vi "LoopselFF_1_or_2cam_eventdriven_HS.VI"() -> ()   [LabVIEW 2015]
uses:
  board.vis/Globals.vi
  <vilib>/Analysis/NI_AALBase.lvlib
panel:
  in  "ADC mode":enum32{"1", "2", "3"}(radio)=enum."3"
  out "tRMS":dbl=8.272957184592048 format="%0#.1f"
  out "mean":dbl=3064.5285285285286 format="%#_4f"
  in  "rms_pixel":u16=100
  in  "continuous":bool=TRUE
  out "curr.block":u8=1
  out "Measure ON":bool
  in  "Board select\n1: board 1\n2: board 2\n3: both boards":u8=3
  in  "no.of blocks (nob)\npress enter":u32=1
  in  "block":u32(slide)=1 max=10 scale=0.9..1.0
  out "Signalverlaufgraph 2":u16[](graph)=[0, 0, 543, 543, 0, 1, 0, 0, 2, 2, 3, 3, 4, 4, 5, 5, 6, 6, 7, 7, 8, 8, 9, 9, 10, 10, 11, 11, 12, 12, 13, 13, 14, 14, 15, 15, 16, 16, 17, 17, 18, 18, 19, 19, 20, 20, 21, 21, 22, 22, 23, 23, 24, 24, 25, 25, 26, 26, 27, 27, 28, 28, 29, 29, 30, 30, 31, 31, 32, 32, 33, 33, 34, 34, 35, 35, 36, 36, 37, 37, 38, 38, 39, 39, 40, 40, 41, 41, 42, 42, 43, 43, 44, 44, 45, 45, 46, 46, 47, 47, 48, 48, 49, 49, 50, 50, 51, 51, 52, 52, 53, 53, 54, 54, 55, 55, 56, 56, 57, 57, 58, 58, 59, 59, 60, 60, 61, 61, 62, 62, 63, 63, 64, 64, 65, 65, 66, 66, 67, 67, 68, 68, 69, 69, 70, 70, 71, 71, 72, 72, 73, 73, 74, 74, 75, 75, 76, 76, 77, 77, 78, 78, 79, 79, 80, 80, 81, 81, 82, 82, 83, 83, 84, 84, 85, 85, 86, 86, 87, 87, 88, 88, 89, 89, 90, 90, 91, 91, 92, 92, 93, 93, 94, 94, 95, 95, 96, 96, 97, 97, 98, 98, 99, 99, 100, 100, 101, 101, 102, 102, 103, 103, 104, 104, 105, 105, 106, 106, 107, 107, 108, 108, 109, 109, 110, 110, 111, 111, 112, 112, 113, 113, 114, 114, 115, 115, 116, 116, 117, 117, 118, 118, 119, 119, 120, 120, 121, 121, 122, 122, 123, 123, 124, 124, 125, 125, 126, 126, 127, 127, 128, 128, 129, 129, 130, 130, 131, 131, 132, 132, 133, 133, 134, 134, 135, 135, 136, 136, 137, 137, 138, 138, 139, 139, 140, 140, 141, 141, 142, 142, 143, 143, 144, 144, 145, 145, 146, 146, 147, 147, 148, 148, 149, 149, 150, 150, 151, 151, 152, 152, 153, 153, 154, 154, 155, 155, 156, 156, 157, 157, 158, 158, 159, 159, 160, 160, 161, 161, 162, 162, 163, 163, 164, 164, 165, 165, 166, 166, 167, 167, 168, 168, 169, 169, 170, 170, 171, 171, 172, 172, 173, 173, 174, 174, 175, 175, 176, 176, 177, 177, 178, 178, 179, 179, 180, 180, 181, 181, 182, 182, 183, 183, 184, 184, 185, 185, 186, 186, 187, 187, 188, 188, 189, 189, 190, 190, 191, 191, 192, 192, 193, 193, 194, 194, 195, 195, 196, 196, 197, 197, 198, 198, 199, 199, 200, 200, 201, 201, 202, 202, 203, 203, 204, 204, 205, 205, 206, 206, 207, 207, 208, 208, 209, 209, 210, 210, 211, 211, 212, 212, 213, 213, 214, 214, 215, 215, 216, 216, 217, 217, 218, 218, 219, 219, 220, 220, 221, 221, 222, 222, 223, 223, 224, 224, 225, 225, 226, 226, 227, 227, 228, 228, 229, 229, 230, 230, 231, 231, 232, 232, 233, 233, 234, 234, 235, 235, 236, 236, 237, 237, 238, 238, 239, 239, 240, 240, 241, 241, 242, 242, 243, 243, 244, 244, 245, 245, 246, 246, 247, 247, 248, 248, 249, 249, 250, 250, 251, 251, 252, 252, 253, 253, 254, 254, 255, 255, 256, 256, 257, 257, 258, 258, 259, 259, 260, 260, 261, 261, 262, 262, 263, 263, 264, 264, 265, 265, 266, 266, 267, 267, 268, 268, 269, 269, 270, 270, 271, 271, 272, 272, 273, 273, 274, 274, 275, 275, 276, 276, 277, 277, 278, 278, 279, 279, 280, 280, 281, 281, 282, 282, 283, 283, 284, 284, 285, 285, 286, 286, 287, 287, 288, 288, 289, 289, 290, 290, 291, 291, 292, 292, 293, 293, 294, 294, 295, 295, 296, 296, 297, 297, 298, 298, 299, 299, 300, 300, 301, 301, 302, 302, 303, 303, 304, 304, 305, 305, 306, 306, 307, 307, 308, 308, 309, 309, 310, 310, 311, 311, 312, 312, 313, 313, 314, 314, 315, 315, 316, 316, 317, 317, 318, 318, 319, 319, 320, 320, 321, 321, 322, 322, 323, 323, 324, 324, 325, 325, 326, 326, 327, 327, 328, 328, 329, 329, 330, 330, 331, 331, 332, 332, 333, 333, 334, 334, 335, 335, 336, 336, 337, 337, 338, 338, 339, 339, 340, 340, 341, 341, 342, 342, 343, 343, 344, 344, 345, 345, 346, 346, 347, 347, 348, 348, 349, 349, 350, 350, 351, 351, 352, 352, 353, 353, 354, 354, 355, 355, 356, 356, 357, 357, 358, 358, 359, 359, 360, 360, 361, 361, 362, 362, 363, 363, 364, 364, 365, 365, 366, 366, 367, 367, 368, 368, 369, 369, 370, 370, 371, 371, 372, 372, 373, 373, 374, 374, 375, 375, 376, 376, 377, 377, 378, 378, 379, 379, 380, 380, 381, 381, 382, 382, 383, 383, 384, 384, 385, 385, 386, 386, 387, 387, 388, 388, 389, 389, 390, 390, 391, 391, 392, 392, 393, 393, 394, 394, 395, 395, 396, 396, 397, 397, 398, 398, 399, 399, 400, 400, 401, 401, 402, 402, 403, 403, 404, 404, 405, 405, 406, 406, 407, 407, 408, 408, 409, 409, 410, 410, 411, 411, 412, 412, 413, 413, 414, 414, 415, 415, 416, 416, 417, 417, 418, 418, 419, 419, 420, 420, 421, 421, 422, 422, 423, 423, 424, 424, 425, 425, 426, 426, 427, 427, 428, 428, 429, 429, 430, 430, 431, 431, 432, 432, 433, 433, 434, 434, 435, 435, 436, 436, 437, 437, 438, 438, 439, 439, 440, 440, 441, 441, 442, 442, 443, 443, 444, 444, 445, 445, 446, 446, 447, 447, 448, 448, 449, 449, 450, 450, 451, 451, 452, 452, 453, 453, 454, 454, 455, 455, 456, 456, 457, 457, 458, 458, 459, 459, 460, 460, 461, 461, 462, 462, 463, 463, 464, 464, 465, 465, 466, 466, 467, 467, 468, 468, 469, 469, 470, 470, 471, 471, 472, 472, 473, 473, 474, 474, 475, 475, 476, 476, 477, 477, 478, 478, 479, 479, 480, 480, 481, 481, 482, 482, 483, 483, 484, 484, 485, 485, 486, 486, 487, 487, 488, 488, 489, 489, 490, 490, 491, 491, 492, 492, 493, 493, 494, 494, 495, 495, 496, 496, 497, 497, 498, 498, 499, 499, 500, 500, 501, 501, 502, 502, 503, 503, 504, 504, 505, 505, 506, 506, 507, 507, 508, 508, 509, 509, 510, 510, 511, 511, 512, 512, 513, 513, 514, 514, 515, 515, 516, 516, 517, 517, 518, 518, 519, 519, 520, 520, 521, 521, 522, 522, 523, 523, 524, 524, 525, 525, 526, 526, 527, 527, 528, 528, 529, 529, 530, 530, 531, 531, 532, 532, 533, 533, 534, 534, 535, 535, 536, 536, 537, 537, 538, 538, 539, 539, 540, 540, 541, 541]
  out "Signalverlaufgraph":u16[](graph)=[2357, 2347, 2353, 2358, 0, 1, 0, 1, 2411, 2350, 2363, 2362, 2360, 34762, 35034, 35066, 35068, 35077, 35067, 35071, 35078, 35087, 35089, 35073, 35080, 35063, 35067, 35068, 35056, 35053, 35026, 35070, 35060, 35052, 35055, 35054, 35023, 35040, 35048, 35039, 35058, 35037, 35044, 35031, 35053, 35025, 35066, 35061, 35050, 35073, 35076, 35083, 35075, 35070, 35075, 35085, 35086, 35080, 35089, 35095, 35070, 35081, 35104, 35104, 35105, 35092, 35088, 35095, 35088, 35081, 35081, 35088, 35080, 35084, 35070, 35082, 35073, 35056, 35058, 35059, 35053, 35054, 35077, 35067, 35059, 35054, 35062, 35059, 35059, 35062, 35066, 35064, 35074, 35065, 35068, 35067, 35064, 35069, 35062, 35075, 35092, 35065, 35066, 35083, 35080, 35080, 35081, 35105, 35099, 35081, 35093, 35095, 35085, 35101, 35101, 35088, 35100, 35088, 35099, 35088, 35085, 35101, 35074, 35079, 35081, 35069, 35058, 35069, 35068, 35075, 35079, 35072, 35080, 35080, 35067, 35078, 35064, 35073, 35063, 35054, 35076, 35075, 35084, 35082, 35085, 35067, 35059, 35082, 35080, 35097, 35083, 35088, 35093, 35097, 35078, 35088, 35097, 35091, 35100, 35088, 35091, 35092, 35100, 35086, 35085, 35097, 35088, 35086, 35079, 35077, 35080, 35089, 35073, 35075, 35083, 35074, 35085, 35070, 35078, 35081, 35070, 35060, 35084, 35077, 35080, 35075, 35069, 35069, 35061, 35065, 35065, 35085, 35071, 35088, 35086, 35088, 35089, 35090, 35091, 35088, 35079, 35100, 35098, 35102, 35082, 35075, 35088, 35079, 35086, 35082, 35098, 35088, 35092, 35085, 35085, 35084, 35097, 35085, 35074, 35072, 35085, 35088, 35079, 35079, 35080, 35085, 35094, 35077, 35090, 35081, 35083, 35089, 35090, 35083, 35083, 35086, 35087, 35083, 35094, 35098, 35093, 35103, 35102, 35089, 35096, 35096, 35078, 35075, 35103, 35084, 35089, 35095, 35093, 35085, 35094, 35090, 35100, 35080, 35099, 35081, 35086, 35095, 35101, 35083, 35090, 35087, 35078, 35096, 35077, 35091, 35102, 35089, 35093, 35100, 35081, 35086, 35088, 35093, 35079, 35088, 35083, 35083, 35100, 35107, 35081, 35096, 35098, 35091, 35098, 35106, 35087, 35107, 35094, 35101, 35099, 35085, 35088, 35093, 35084, 35089, 35100, 35096, 35094, 35099, 35085, 35094, 35089, 35104, 35088, 35103, 35099, 35088, 35088, 35083, 35092, 35097, 35096, 35095, 35098, 35076, 35100, 35091, 35084, 35090, 35100, 35110, 35101, 35071, 35094, 35088, 35097, 35076, 35103, 35100, 35102, 35101, 35094, 35096, 35103, 35088, 35093, 35099, 35099, 35102, 35099, 35104, 35089, 35085, 35094, 35110, 35093, 35109, 35094, 35101, 35088, 35100, 35090, 35088, 35090, 35086, 35093, 35107, 35091, 35099, 35104, 35088, 35093, 35093, 35098, 35097, 35108, 35087, 35107, 35092, 35094, 35098, 35097, 35092, 35093, 35085, 35095, 35102, 35094, 35093, 35115, 35088, 35106, 35079, 35105, 35099, 35091, 35128, 35094, 35089, 35088, 35109, 35110, 35087, 35110, 35096, 35095, 35097, 35091, 35099, 35085, 35087, 35112, 35089, 35102, 35085, 35089, 35106, 35094, 35097, 35113, 35110, 35087, 35105, 35097, 35094, 35097, 35097, 35098, 35112, 35092, 35101, 35106, 35092, 35094, 35085, 35107, 35088, 35089, 35094, 35081, 35094, 35103, 35107, 35097, 35101, 35086, 35094, 35108, 35086, 35098, 35102, 35102, 35096, 35080, 35085, 35100, 35089, 35088, 35104, 35112, 35100, 35102, 35102, 35097, 35106, 35099, 35081, 35097, 35101, 35109, 35100, 35114, 35098, 35092, 32940, 29697, 29585, 29528, 29434, 29346, 29303, 29248, 29143, 29102, 29112, 29035, 28966, 28956, 28848, 28789, 28725, 28651, 28612, 28562, 28516, 28427, 28371, 28320, 28264, 28200, 28178, 28101, 28056, 27957, 27925, 27901, 27776, 27758, 27701, 27631, 27579, 27545, 27475, 27425, 27382, 27318, 27302, 27222, 27176, 27114, 27069, 27020, 26974, 26944, 26887, 26793, 26807, 26744, 26714, 26624, 26586, 26540, 26466, 26393, 26379, 26282, 26220, 26157, 26029, 25929, 25768, 25543, 2252, 2400, 2386, 2390, 2368, 2373, 2377, 2379, 2379, 2378, 2377, 2380, 2373, 2379, 2386, 2383, 2376, 2381, 2378, 2377, 2376, 2373, 2385, 2377, 2381, 2376, 2379, 2379, 2376, 2376, 2376, 2379, 2384, 2378, 2374, 2380, 2377, 2381, 2380, 2371, 2379, 2376, 2379, 2384, 2380, 2380, 2377, 2368, 2376, 2375, 2378, 2370, 2374, 2375, 2383, 2372, 2379, 2374, 2381, 2369, 2375, 2368, 2373, 2368, 2368, 2372, 2374, 2371, 2368, 2373, 2372, 2370, 2372, 2374, 2375, 2367, 2367, 2370, 2369, 2375, 2372, 2373, 2378, 2372, 2366, 2372, 2370, 2374, 2365, 2373, 2375, 2374, 2370, 2370, 2369, 2369, 2374, 2371, 2373, 2371, 2372, 2371, 2366, 2368, 2370, 2362, 2370, 2372, 2366, 2374, 2369, 2368, 2371, 2368, 2365, 2362, 2375, 2373, 2369, 2366, 2367, 2371, 2362, 2377, 2371, 2367, 2369, 2366, 2371, 2366, 2364, 2366, 2360, 2365, 2374, 2362, 2371, 2373, 2366, 2364, 2367, 2364, 2368, 2360, 2360, 2363, 2367, 2368, 2367, 2371, 2364, 2368, 2366, 2359, 2363, 2365, 2368, 2368, 2358, 2357, 2365, 2364, 2369, 2362, 2364, 2364, 2363, 2358, 2363, 2364, 2359, 2360, 2358, 2370, 2358, 2361, 2363, 2355, 2361, 2369, 2363, 2366, 2365, 2368, 2363, 2360, 2359, 2361, 2359, 2363, 2356, 2365, 2362, 2360, 2368, 2362, 2366, 2370, 2358, 2366, 2364, 2366, 2362, 2363, 2356, 2365, 2363, 2361, 2363, 2367, 2366, 2365, 2357, 2366, 2359, 2361, 2360, 2360, 2363, 2365, 2364, 2360, 2360, 2357, 2355, 2362, 2361, 2361, 2364, 2364, 2361, 2364, 2361, 2363, 2358, 2363, 2357, 2355, 2357, 2365, 2357, 2367, 2365, 2363, 2354, 2360, 2356, 2358, 2362, 2359, 2360, 2362, 2362, 2355, 2360, 2360, 2360, 2361, 2360, 2359, 2357, 2364, 2359, 2361, 2362, 2360, 2359, 2360, 2355, 2355, 2362, 2358, 2358, 2357, 2357, 2360, 2360, 2363, 2353, 2353, 2358, 2358, 2358, 2362, 2360, 2362, 2359, 2356, 2357, 2360, 2355, 2353, 2360, 2362, 2358, 2358, 2350, 2357, 2362, 2354, 2354, 2356, 2360, 2360, 2355, 2361, 2354, 2360, 2356, 2355, 2355, 2362, 2359, 2362, 2363, 2359, 2361, 2358, 2355, 2356, 2354, 2358, 2364, 2356, 2362, 2358, 2354, 2360, 2362, 2361, 2358, 2361, 2362, 2358, 2363, 2359, 2363, 2364, 2356, 2357, 2356, 2354, 2360, 2357, 2355, 2359, 2358, 2356, 2362, 2360, 2357, 2359, 2357, 2357, 2355, 2357, 2357, 2357, 2364, 2360, 2355, 2358, 2355, 2357, 2360, 2353, 2355, 2352, 2362, 2354, 2355, 2360, 2357, 2352, 2359, 2356, 2356, 2358, 2353, 2357, 2356, 2355, 2349, 2361, 2358, 2354, 2358, 2359, 2355, 2360, 2354, 2357, 2357, 2353, 2354, 2359, 2359, 2355, 2349, 2358, 2358, 2355, 2353, 2353, 2357, 2357, 2357, 2354, 2358, 2359, 2354, 2353, 2352, 2358, 2361, 2357, 2350, 2350, 2352, 2360, 2351, 2355, 2354, 2360, 2357, 2355, 2355, 2355, 2350, 2357, 2357, 2358, 2358, 2356, 2353, 2352, 2354, 2353, 2357, 2357, 2353, 2358, 2360, 2361, 2355, 2357, 2361, 2357, 2358, 2356, 2355, 2358, 2354, 2351, 2355, 2352, 2354, 2352, 2354, 2363, 2359, 2358, 2357, 2349, 2358, 2352, 2356, 2355, 2359, 2353, 2353, 2361, 2359, 2359, 2357, 2357, 2349, 2353, 2353, 2350, 2358, 2357, 2356, 2358, 2356, 2356, 2355, 2355, 2355, 2351, 2355, 2357, 2352, 2354, 2348, 2354, 2348, 2354, 2350, 2352, 2353, 2359, 2356, 2351, 2356, 2357, 2352, 2354, 2355, 2359, 2353, 2354, 2352, 2349, 2362, 2353, 2360, 2349, 2357, 2352, 2359, 2348, 2359, 2349, 2358, 2348, 2349, 2351, 2356, 2353, 2358, 2353, 2354, 2360, 2355, 2356, 2358, 2348, 2351, 2354, 2358, 2360, 2360, 2359, 2356, 2356, 2354, 2357, 2350, 2351, 2351]
  out "boards recognised":u8=1
  in  "alloc mem":bool
  out "FREE \nRAM MB":dbl=14941.0
  out "BUILT-IN\nRAM MB":dbl=18096.0
  out "SEC":dbl=5.9999999999999995e-05
  out "MB RAM":dbl
  in  "pos slope":u8=1
  in  "both slopes":u8
  in  "DAT in 10ns":u32
  in  "extTrig  0/1\n0 : internal\n1:  \"I\" input (laser)":u8
  in  "stop all":bool
  in  "start":bool
  in  "sample":u32(slide)=2 max=3000 scale=0.9..110.0
  in  "no.of samples (nos)":u32=3000
  in  "exposuretime[ms]":dbl=1.0 format="%.3f"
  # "Start with run"
  # "Abort with ESC"
  # "press Esc to stop measurement"
  # "exit here"
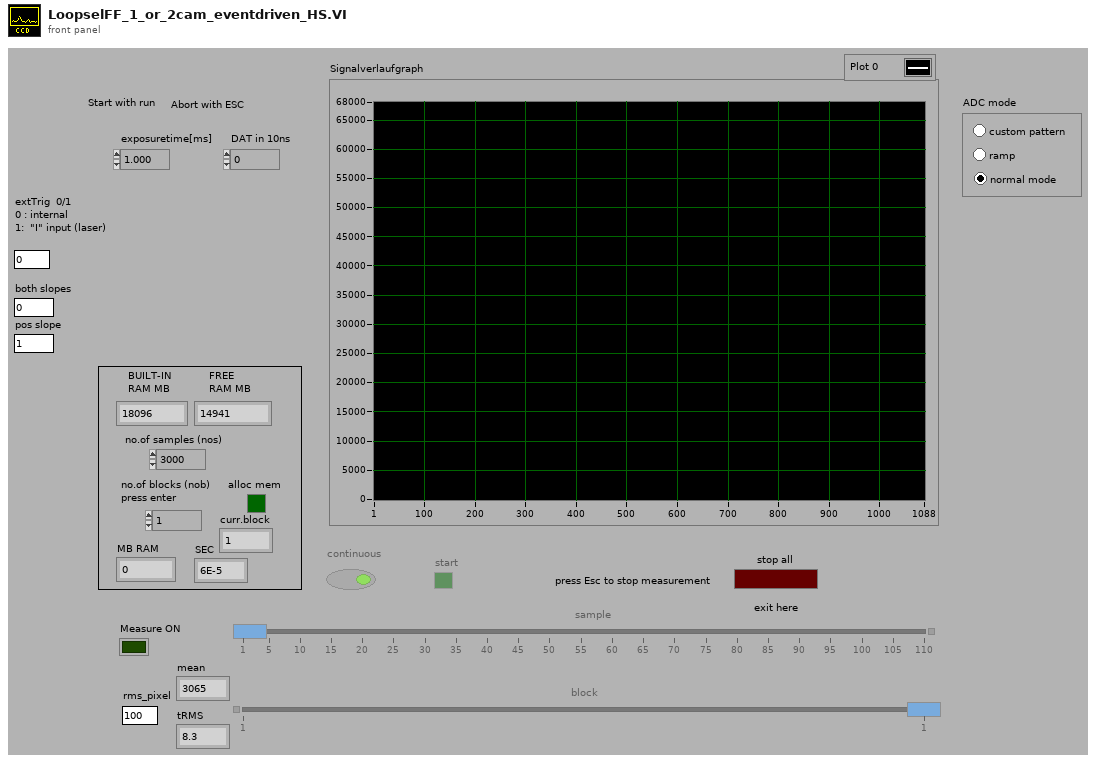
[diagram p1: front panel]
types:
  T1 = enum8{"Enabled", "Disabled", "Disabled and Grayed Out"}
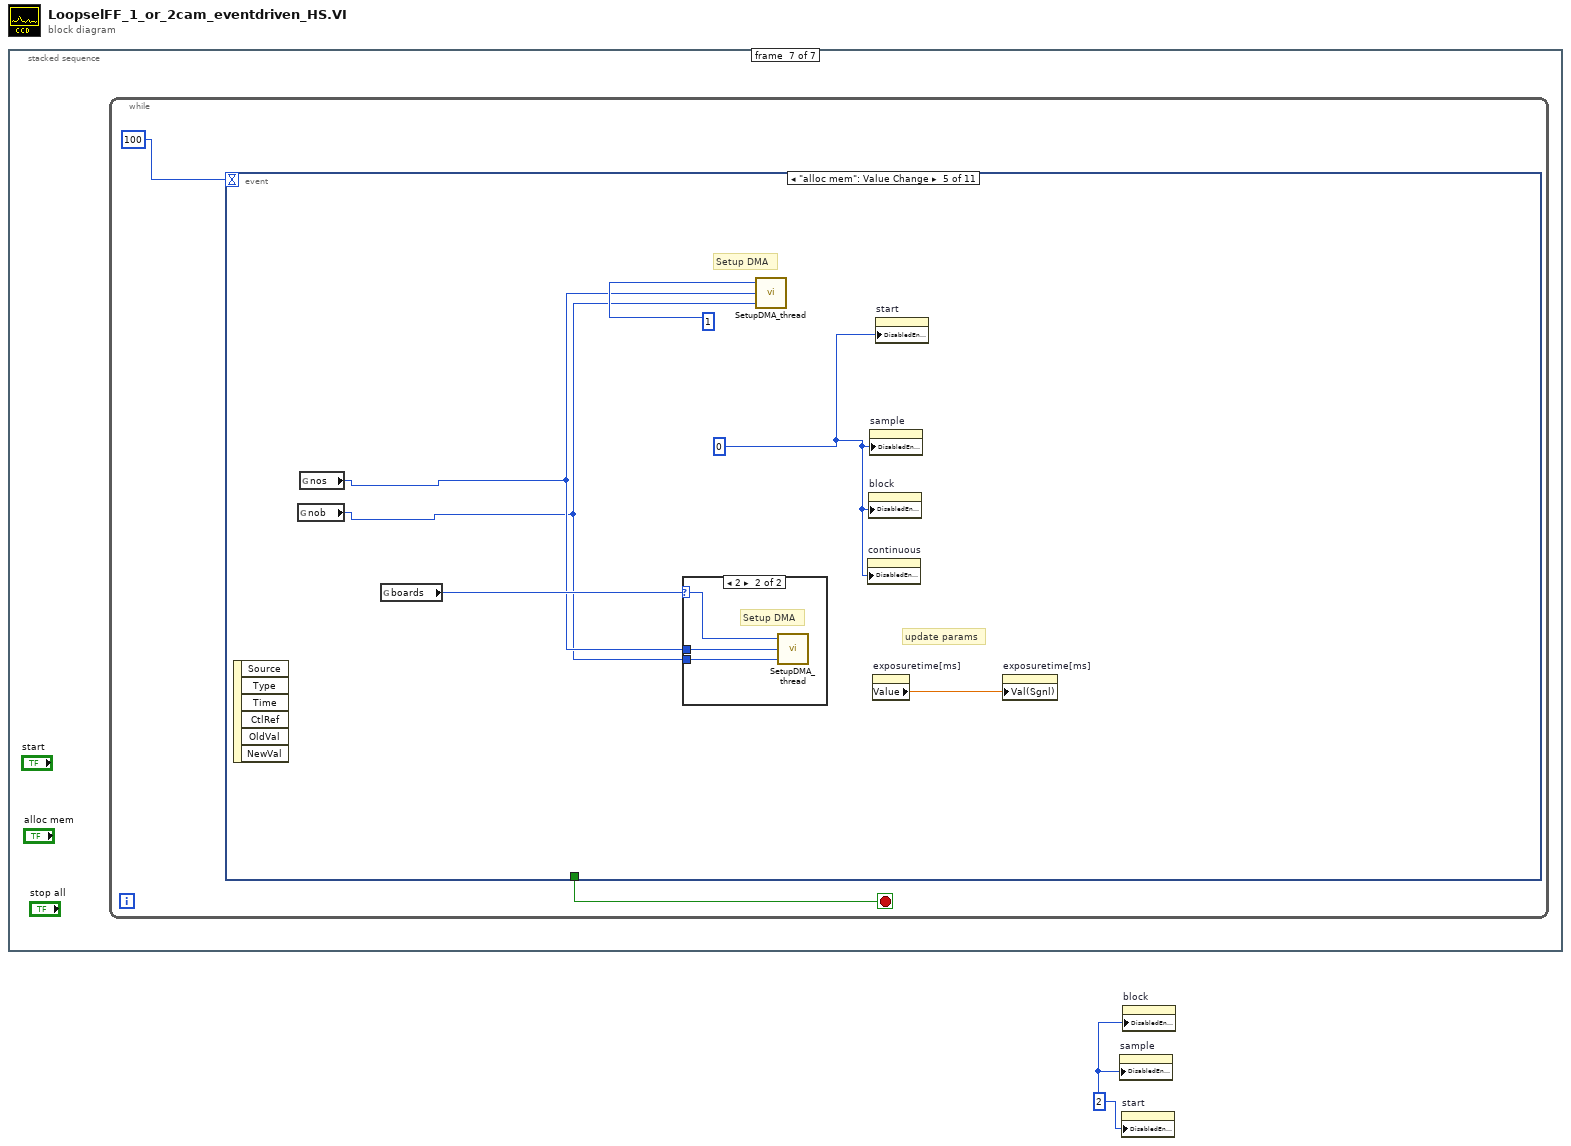
[diagram p0: block diagram]
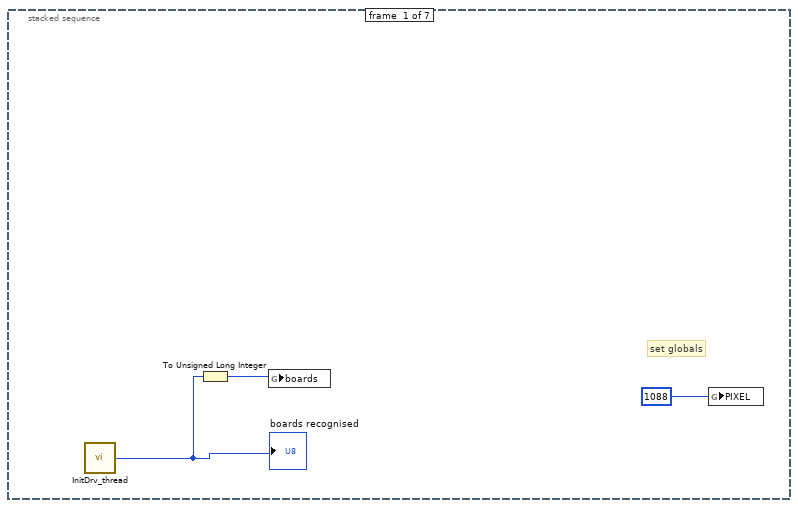
[diagram p2: hidden frame]
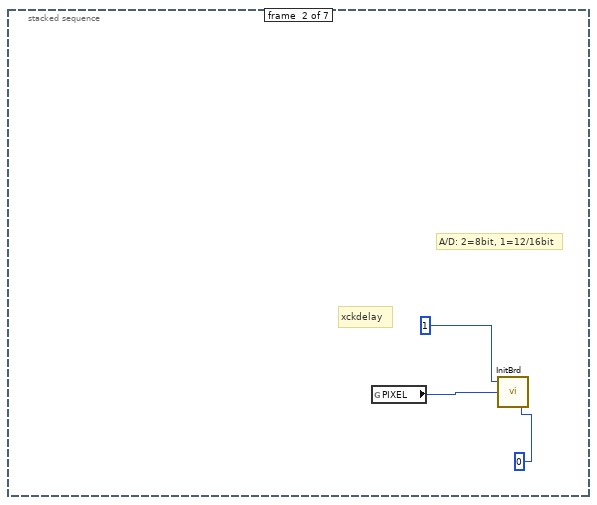
[diagram p3: hidden frame]
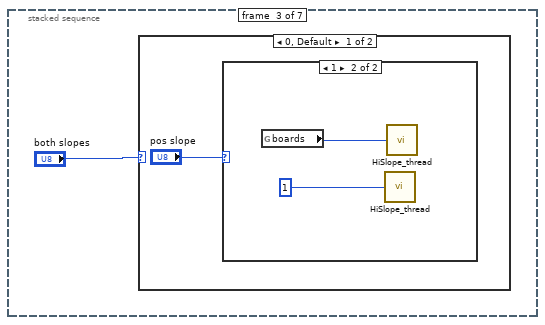
[diagram p4: hidden frame]
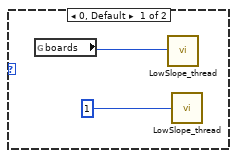
[diagram p5: hidden frame]
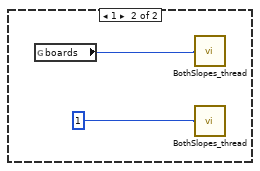
[diagram p6: hidden frame]
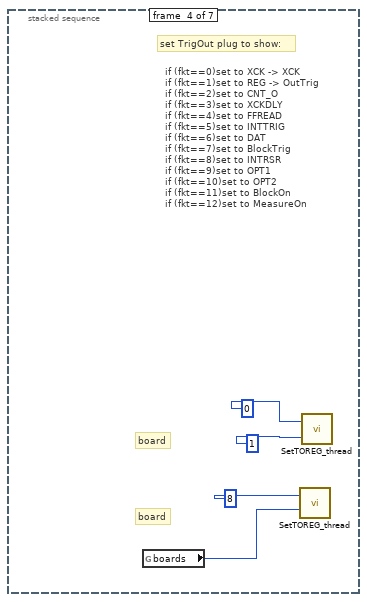
[diagram p7: hidden frame]
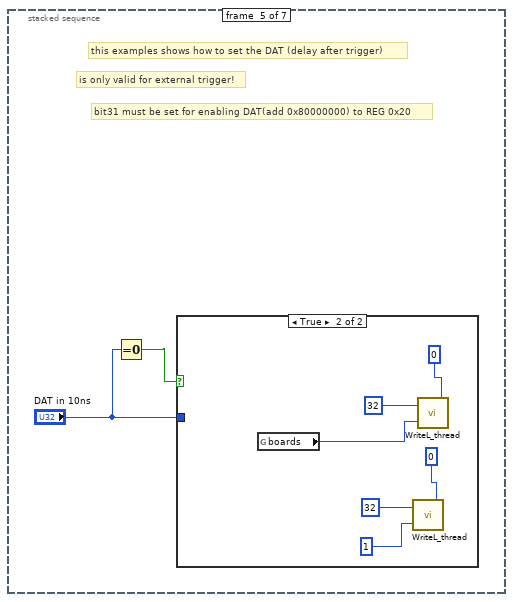
[diagram p8: hidden frame]
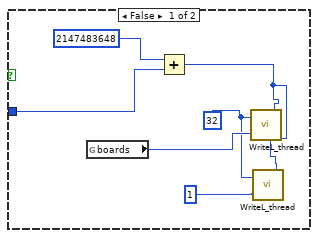
[diagram p9: hidden frame]
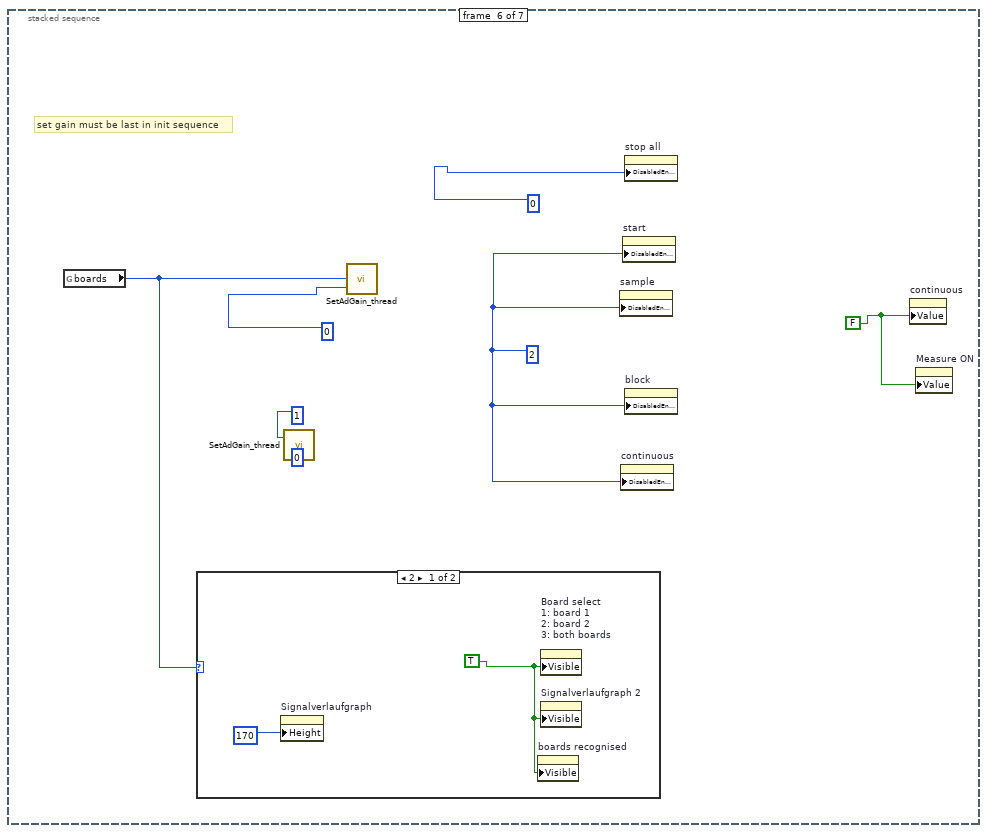
[diagram p10: hidden frame]
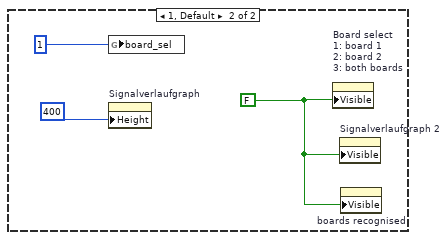
[diagram p11: hidden frame]
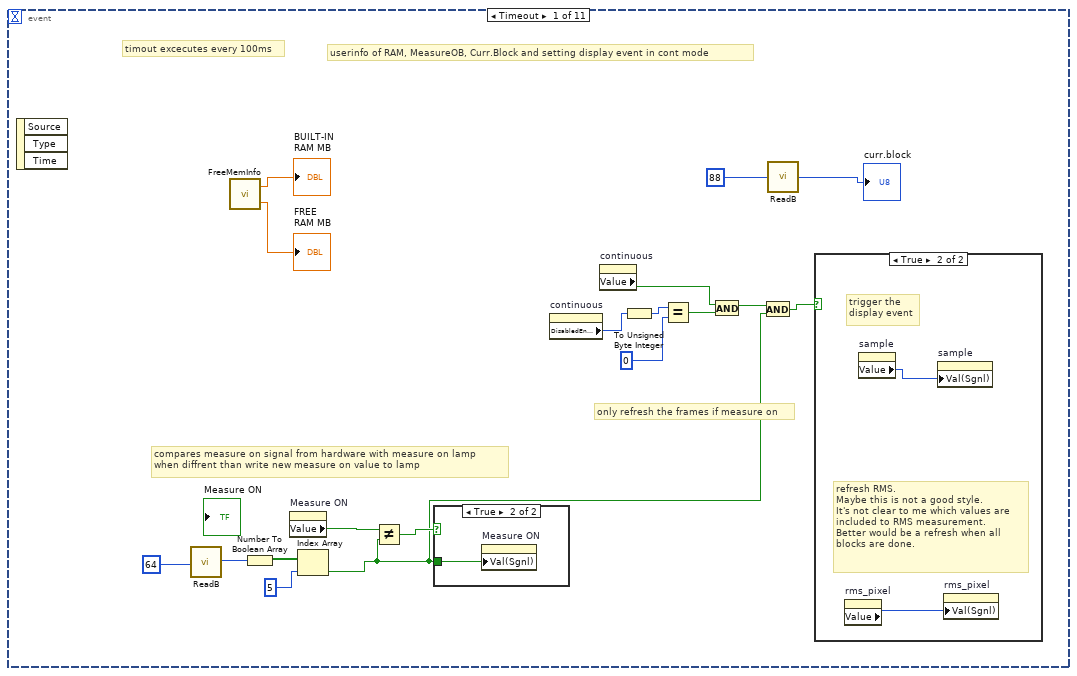
[diagram p12: hidden frame]
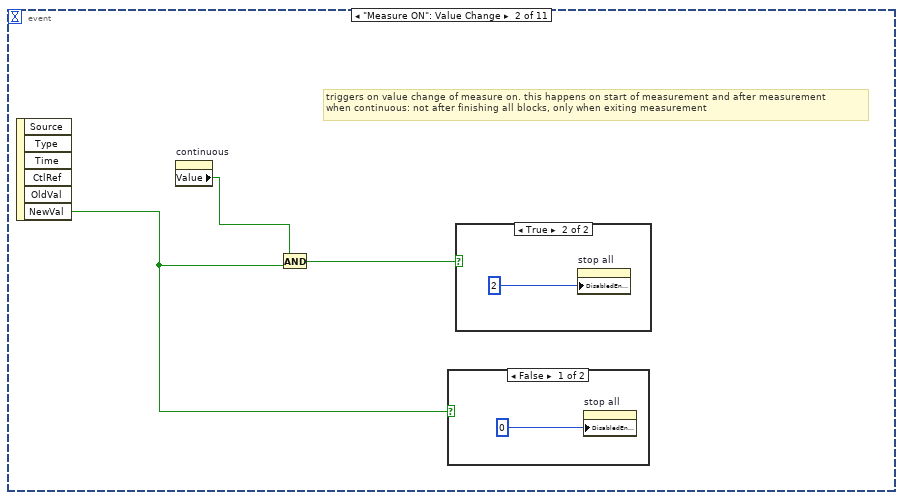
[diagram p15: hidden frame]
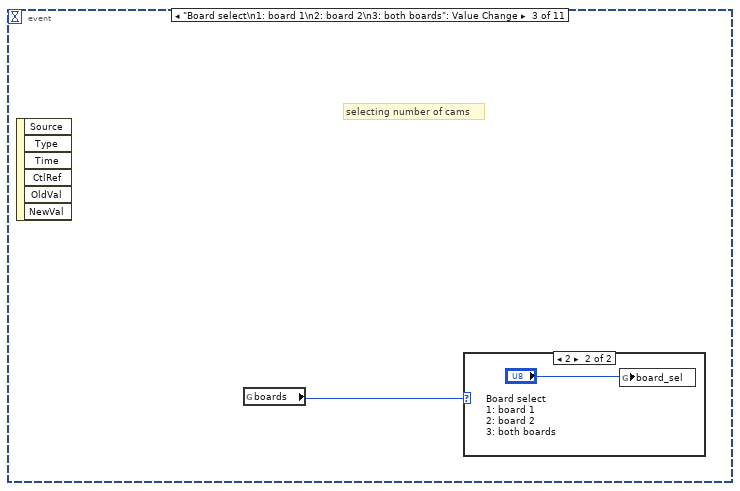
[diagram p18: hidden frame]
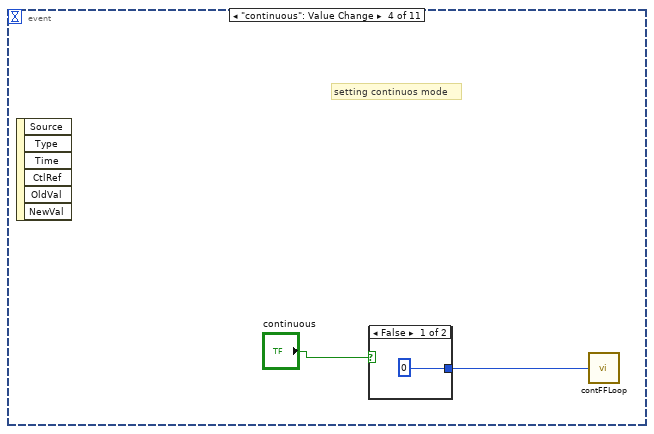
[diagram p20: hidden frame]
diagram:
  w1 = 2
  n1 = stacked-sequence {
    frame #0 {
      # "set globals"
      n2 = call "InitDrv_thread.vi"() -> ("Boards"=w2:u8)  [unwired: 1 in]
      "boards recognised" <- w2
      n3 = To Unsigned Long Integer(number=w2) -> (unsigned 32bit integer=w3:u32)
      n4 = global write "Globals.vi" "boards"(w3) -> ()
      n5 = global write "Globals.vi" "PIXEL"(u32 1088) -> ()
    }
    frame #1 {
      # "xckdelay"
      # "A/D: 2=8bit, 1=12/16bit"
      n6 = global read "Globals.vi" "PIXEL"() -> (w7:u32)
      n7 = call "InitBrd.vi"("xckdly"=u32 0, "pixel"=w7, "flag816"=u32 1) -> ()  [unwired: 3 in]
    }
    frame #2 {
      n8 = case shown="0, Default" "both slopes" {
        frame 0, Default {
          n9 = case shown="1" "pos slope" {
            frame 0, Default {
              n10 = global read "Globals.vi" "boards"() -> (w10:u32)
              n11 = call "LowSlope_thread.vi"("board"=w10) -> ()  [unwired: 1 in]
              n12 = call "LowSlope_thread.vi"("board"=u32 1) -> ()  [unwired: 1 in]
            }
            frame 1 {
              n13 = global read "Globals.vi" "boards"() -> (w13:u32)
              n14 = call "HiSlope_thread.vi"("board"=u32 1) -> ()  [unwired: 1 in]
              n15 = call "HiSlope_thread.vi"("board"=w13) -> ()  [unwired: 1 in]
            }
          }
        }
        frame 1 {
          n16 = global read "Globals.vi" "boards"() -> (w15:u32)
          n17 = call "BothSlopes_thread.vi"("board"=w15) -> ()  [unwired: 1 in]
          n18 = call "BothSlopes_thread.vi"("board"=u32 1) -> ()  [unwired: 1 in]
        }
      }
    }
    frame #3 {
      # "board"
      # "board"
      # "set TrigOut plug to show:"
      # "if (fkt==0)set to XCK -> XCK\nif (fkt==1)set to REG -> OutTrig\nif (fkt==2)set to CNT_O\nif (fkt==3)set to XCKDLY\nif (fkt==4)set to FFREAD\nif (fkt==5)set to INTTRIG\nif (fkt==6)set to DAT\nif (fkt==7)set to BlockTrig\nif (fkt==8)set to INTRSR\nif (fkt==9)set to OPT1\nif (fkt==10)set to OPT2\nif (fkt==11)set to BlockOn\nif (fkt==12)set to MeasureOn"
      n19 = global read "Globals.vi" "boards"() -> (w19:u32)
      n20 = call "SetTOREG_thread.vi"("board"=w19, "fkt"=u8 8) -> ()  [unwired: 1 in]
      n21 = call "SetTOREG_thread.vi"("board"=u32 1, "fkt"=u8 0) -> ()  [unwired: 1 in]
    }
    frame #4 {
      # "bit31 must be set for enabling DAT(add 0x80000000) to REG 0x20"
      # "is only valid for external trigger!"
      # "this examples shows how to set the DAT (delay after trigger)"
      n22 = Equal To 0?(x="DAT in 10ns") -> (x = 0?=w21:bool)
      n23 = case shown="True" w21 {
        tunnel: "DAT in 10ns" -> [w26 _]
        frame False {
          w23 = u32 32
          n24 = global read "Globals.vi" "boards"() -> (w25:u32)
          n25 = Add(x=u32 2147483648, y=w26) -> (x+y=w24:u32)
          n26 = call "WriteL_thread.vi"("val"=w24, "board"=w25, "offset"=w23) -> ()
          n27 = call "WriteL_thread.vi"("val"=w24, "board"=u32 1, "offset"=w23) -> ()
        }
        frame True {
          n28 = global read "Globals.vi" "boards"() -> (w32:u32)
          n29 = call "WriteL_thread.vi"("val"=u32 0, "board"=u32 1, "offset"=u32 32) -> ()
          n30 = call "WriteL_thread.vi"("val"=u32 0, "board"=w32, "offset"=u32 32) -> ()
        }
      }
    }
    frame #5 {
      w34 = FALSE
      w40 = 2
      # "set gain must be last in init sequence"
      n31 = global read "Globals.vi" "boards"() -> (w38:u32)
      n32 = case shown="2" w38 {
        frame 2 {
          w42 = TRUE
          n33 = property on="Signalverlaufgraph" class="WFGraph (strict)"("Height"=u8 170) -> ()  [unwired: 2 in, 2 out]
          n34 = property on="boards recognised" class="DigNum (strict)"("Visible"=w42) -> ()  [unwired: 2 in, 2 out]
          n35 = property on="Board select\n1: board 1\n2: board 2\n3: both boards" class="DigNum (strict)"("Visible"=w42) -> ()  [unwired: 2 in, 2 out]
          n36 = property on="Signalverlaufgraph 2" class="WFGraph (strict)"("Visible"=w42) -> ()  [unwired: 2 in, 2 out]
        }
        frame 1, Default {
          w43 = FALSE
          n37 = global write "Globals.vi" "board_sel"(u8 1) -> ()
          n38 = property on="Signalverlaufgraph" class="WFGraph (strict)"("Height"=400) -> ()  [unwired: 2 in, 2 out]
          n39 = property on="Board select\n1: board 1\n2: board 2\n3: both boards" class="DigNum (strict)"("Visible"=w43) -> ()  [unwired: 2 in, 2 out]
          n40 = property on="Signalverlaufgraph 2" class="WFGraph (strict)"("Visible"=w43) -> ()  [unwired: 2 in, 2 out]
          n41 = property on="boards recognised" class="DigNum (strict)"("Visible"=w43) -> ()  [unwired: 2 in, 2 out]
        }
      }
      n42 = call "SetAdGain_thread.vi"("gain"=u8 0, "board"=u32 1) -> ()  [unwired: 1 in]
      n43 = call "SetAdGain_thread.vi"("gain"=u8 0, "board"=w38) -> ()  [unwired: 1 in]
      n44 = property on="sample" class="Slide (strict)"("DisabledEnum"=w40) -> ()  [unwired: 2 in, 2 out]
      n45 = property on="continuous" class="Bool (strict)"("DisabledEnum"=w40) -> ()  [unwired: 2 in, 2 out]
      n46 = property on="start" class="Bool (strict)"("DisabledEnum"=w40) -> ()  [unwired: 2 in, 2 out]
      n47 = property on="stop all" class="Bool (strict)"("DisabledEnum"=0) -> ()  [unwired: 2 in, 2 out]
      n48 = property on="block" class="Slide (strict)"("DisabledEnum"=w40) -> ()  [unwired: 2 in, 2 out]
      n49 = property on="continuous" class="Bool (strict)"("Value"=w34) -> ()  [unwired: 2 in, 2 out]
      n50 = property on="Measure ON" class="Bool (strict)"("Value"=w34) -> ()  [unwired: 2 in, 2 out]
    }
    frame #6 {
      n51 = while {
        stop <- w47 stop-if-true
        n52 = event shown="[4] \"alloc mem\": Value Change" {
          selector: _ -> [_ _ _ _ _ _ _ _ _ _ _]
          dyn-events: _ -> [_ _ _ _ _ _ _ _ _ _ _]
          timeout: 100 -> [_ _ _ _ _ _ _ _ _ _ _]
          tunnel: [_ _ _ _ _ _ _ _ w153 _ _] -> w47
          event Timeout {
            # "only refresh the frames if measure on"
            # "compares measure on signal from hardware with measure on lamp\nwhen diffrent than write new measure on value to lamp"
            # "timout excecutes every 100ms"
            # "userinfo of RAM, MeasureOB, Curr.Block and setting display event in cont mode"
            n53 = event-data() -> ()  [unwired: 1 in, 3 out]
            n54 = call "ReadB.vi"("Offset"=u32 64) -> ("Data"=w62:u8)
            n55 = call "FreeMemInfo.vi"() -> ("PhysicalSpace"=→"BUILT-IN\nRAM MB":dbl, "PhysicalFreeSpace"=→"FREE \nRAM MB":dbl)  [unwired: 1 in]
            n56 = Number To Boolean Array(number=w62) -> (Boolean array=w61:bool[])
            n57 = property on="Measure ON" class="Bool (strict)"() -> ("Value"=w55:bool)  [unwired: 2 in, 2 out]
            n58 = Index Array(array=w61, index=5) -> (element=w51:bool)
            n59 = Not Equal?(x=w55, y=w51) -> (x != y?=w54:bool)
            n60 = case shown="True" w54 {
              tunnel: w51 -> [_ w66]
              frame False {
              }
              frame True {
                n61 = property on="Measure ON" class="Bool (strict)"("Val(Sgnl)"=w66) -> ()  [unwired: 2 in, 2 out]
              }
            }
            n62 = property on="continuous" class="Bool (strict)"() -> ("DisabledEnum"=w48:T1)  [unwired: 2 in, 2 out]
            n63 = property on="continuous" class="Bool (strict)"() -> ("Value"=w57:bool)  [unwired: 2 in, 2 out]
            n64 = To Unsigned Byte Integer(number=w48) -> (unsigned 8bit integer=w49:u8)
            n65 = Equal?(x=w49, y=u8 0) -> (x = y?=w56:bool)
            n66 = And(x=w57, y=w56) -> (x .and. y?=w53:bool)
            n67 = And(x=w53, y=w51) -> (x .and. y?=w52:bool)
            n68 = call "ReadB.vi"("Offset"=u32 88) -> ("Data"=→"curr.block":u8)
            n69 = case shown="True" w52 {
              frame False {
              }
              frame True {
                # "refresh RMS.\nMaybe this is not a good style.\nIt's not clear to me which values are \nincluded to RMS measurement.\nBetter would be a refresh when all\nblocks are done."
                # "trigger the \ndisplay event"
                n70 = property on="rms_pixel" class="DigNum (strict)"() -> ("Value"=w67:u16)  [unwired: 2 in, 2 out]
                n71 = property on="sample" class="Slide (strict)"() -> ("Value"=w68:u32)  [unwired: 2 in, 2 out]
                n72 = property on="sample" class="Slide (strict)"("Val(Sgnl)"=w68) -> ()  [unwired: 2 in, 2 out]
                n73 = property on="rms_pixel" class="DigNum (strict)"("Val(Sgnl)"=w67) -> ()  [unwired: 2 in, 2 out]
              }
            }
          }
          event "Measure ON": Value Change {
            # "triggers on value change of measure on. this happens on start of measurement and after measurement\nwhen continuous: not after finishing all blocks, only when exiting measurement"
            n74 = event-data() -> ("NewVal"=w69:bool)  [unwired: 1 in, 5 out]
            n75 = property on="continuous" class="Bool (strict)"() -> ("Value"=w70:bool)  [unwired: 2 in, 2 out]
            n76 = And(x=w70, y=w69) -> (x .and. y?=w71:bool)
            n77 = case shown="False" w69 {
              frame False {
                n78 = property on="stop all" class="Bool (strict)"("DisabledEnum"=0) -> ()  [unwired: 2 in, 2 out]
              }
              frame True {
              }
            }
            n79 = case shown="True" w71 {
              frame False {
              }
              frame True {
                n80 = property on="stop all" class="Bool (strict)"("DisabledEnum"=2) -> ()  [unwired: 2 in, 2 out]
              }
            }
          }
          event "Board select\n1: board 1\n2: board 2\n3: both boards": Value Change {
            # "selecting number of cams"
            n81 = event-data() -> ()  [unwired: 1 in, 6 out]
            n82 = global read "Globals.vi" "boards"() -> (w74:u32)
            n83 = case shown="2" w74 {
              frame 0, Default {
              }
              frame 2 {
                n84 = global write "Globals.vi" "board_sel"("Board select\n1: board 1\n2: board 2\n3: both boards") -> ()
              }
            }
          }
          event "continuous": Value Change {
            # "setting continuos mode"
            n85 = event-data() -> ()  [unwired: 1 in, 6 out]
            n86 = case shown="False" "continuous" {
              tunnel: [u8 0 u8 1] -> w76
              frame False {
              }
              frame True {
              }
            }
            n87 = call "contFFLoop.vi"("Numeric"=w76) -> ()  [unwired: 1 in]
          }
          event "alloc mem": Value Change {
            w82 = 0
            # "update params"
            # "Setup DMA"
            n88 = event-data() -> ()  [unwired: 1 in, 6 out]
            n89 = global read "Globals.vi" "nob"() -> (w80:u32)
            n90 = global read "Globals.vi" "nos"() -> (w81:u32)
            n91 = global read "Globals.vi" "boards"() -> (w85:u32)
            n92 = case shown="2" w85 {
              selector: w85 -> [_ w86]
              tunnel: w81 -> [_ w87]
              tunnel: w80 -> [_ w88]
              frame 1, Default {
              }
              frame 2 {
                # "Setup DMA"
                n93 = call "SetupDMA_thread.vi"("blocks"=w88, "nos"=w87, "Drv"=w86) -> ()  [unwired: 2 in]
              }
            }
            n94 = call "SetupDMA_thread.vi"("blocks"=w80, "nos"=w81, "Drv"=u32 1) -> ()  [unwired: 2 in]
            n95 = property on="continuous" class="Bool (strict)"("DisabledEnum"=w82) -> ()  [unwired: 2 in, 2 out]
            n96 = property on="block" class="Slide (strict)"("DisabledEnum"=w82) -> ()  [unwired: 2 in, 2 out]
            n97 = property on="sample" class="Slide (strict)"("DisabledEnum"=w82) -> ()  [unwired: 2 in, 2 out]
            n98 = property on="exposuretime[ms]" class="DigNum (strict)"() -> ("Value"=w84:dbl)  [unwired: 2 in, 2 out]
            n99 = property on="start" class="Bool (strict)"("DisabledEnum"=w82) -> ()  [unwired: 2 in, 2 out]
            n100 = property on="exposuretime[ms]" class="DigNum (strict)"("Val(Sgnl)"=w84) -> ()  [unwired: 2 in, 2 out]
          }
          event "start": Mouse Down {
            # "start measurement"
            # "only 1st PCI board is used for ext. trig."
            # "ext. block trig\n0: internal: Space\n1: PCI \"I\"\n2: S1\n3: S2"
            # "block trigger 0/1\n0: internal -> next block is started immediately \n1: external -> each block has an own trigger"
            n101 = event-data() -> ()  [unwired: 1 in, 8 out]
            n102 = global read "Globals.vi" "exp time"() -> (w94:dbl)
            n103 = Multiply(x=1000.0, y=w94) -> (x*y=w96:dbl)
            n104 = global read "Globals.vi" "board_sel"() -> (w89:u8)
            n105 = To Unsigned Long Integer(number=w96) -> (unsigned 32bit integer=w91:u32)
            n106 = call "ReadFFLoop_thread.vi"("blocktrigger"=u8 0, "btrig_ch"=u8 0, "ExtTrig"="extTrig  0/1\n0 : internal\n1:  \"I\" input (laser)", "cam_sel"=w89, "exptus"=w91) -> ()  [unwired: 1 in]
          }
          event "sample", "block": Value Change {
            w108 = u32 1
            # "when selecting a value\nbigger than possible\nnos or nob, a dummy \nvalue \"1\" is chosen\n\nTODO:\ninsert error handling\nwith lower values than 1"
            # "display"
            n107 = event-data() -> ()  [unwired: 1 in, 6 out]
            n108 = global read "Globals.vi" "boards"() -> (w111:u32)
            n109 = global read "Globals.vi" "nob"() -> (w100:u32)
            n110 = global read "Globals.vi" "nos"() -> (w107:u32)
            n111 = Greater?(x=w100, y="block") -> (0:w103:bool)
            n112 = Greater?(x=w107, y="sample") -> (0:w106:bool)
            n113 = global read "Globals.vi" "PIXEL"() -> (w97:u32)
            n114 = case shown="False" w103 {
              tunnel: [u32 1 w116] -> w102
              tunnel: "block" -> [_ w116]
              frame False {
              }
              frame True {
              }
            }
            n115 = case shown="False" w106 {
              tunnel: [u32 1 w118] -> w105
              tunnel: "sample" -> [_ w118]
              frame False {
              }
              frame True {
              }
            }
            n116 = To Long Integer(number=w97) -> (32bit integer=w98:i32)
            n117 = Initialize Array(u16 100, w98) -> (w114:u16[])
            n118 = Subtract(x=w105, y=w108) -> (x-y=w110:u32)
            n119 = Subtract(x=w102, y=w108) -> (x-y=w109:u32)
            n120 = case shown="2" w111 {
              selector: w111 -> [_ w123]
              tunnel: w110 -> [_ w124]
              tunnel: w109 -> [_ w121]
              frame 0, Default {
              }
              frame 2 {
                n121 = global read "Globals.vi" "PIXEL"() -> (w119:u32)
                n122 = To Long Integer(number=w119) -> (32bit integer=w120:i32)
                n123 = Initialize Array(u16 100, w120) -> (w126:u16[])
                n124 = call "ReturnFrame.vi"("Data Values In"=w126, "curr_nob"=w121, "curr_nos"=w124, "Drv"=w123) -> ("Data Values Out"=→"Signalverlaufgraph 2":u16[])  [unwired: 1 in]
              }
            }
            n125 = call "ReturnFrame.vi"("Data Values In"=w114, "curr_nob"=w109, "curr_nos"=w110, "Drv"=u32 1) -> ("Data Values Out"=→"Signalverlaufgraph":u16[])  [unwired: 1 in]
          }
          event "no.of samples (nos)", "no.of blocks (nob)\npress enter", "exposuretime[ms]": Value Change {
            # "calculation of MB RAM an SEC and setting scale max"
            # "MB"
            # "ushort"
            n126 = event-data() -> ()  [unwired: 1 in, 7 out]
            n127 = global read "Globals.vi" "PIXEL"() -> (w152:u32)
            n128 = Multiply(x="no.of samples (nos)", y=w152) -> (x*y=w150:u32)
            n129 = Multiply(x=w150, y=u32 2) -> (x*y=w130:u32)
            n130 = global read "Globals.vi" "boards"() -> (w151:u32)
            n131 = global read "Globals.vi" "cams_amount"() -> (w129:u8)
            n132 = global read "Globals.vi" "nos"() -> (w134:u32)
            n133 = global read "Globals.vi" "nob"() -> (w132:u32)
            n134 = To Unsigned Long Integer(number=w129) -> (unsigned 32bit integer=w128:u32)
            n135 = Multiply(x=w128, y=w130) -> (x*y=w127:u32)
            n136 = Multiply(x=w127, y=w151) -> (x*y=w140:u32)
            n137 = To Double Precision Float(number=w140) -> (double precision float=w139:dbl)
            n138 = To Double Precision Float(number=w134) -> (double precision float=w133:dbl)
            n139 = Divide(x=w139, y=1048576.0) -> (x/y=w142:dbl)
            n140 = To Double Precision Float(number=w132) -> (double precision float=w131:dbl)
            n141 = To Double Precision Float(number="no.of blocks (nob)\npress enter") -> (double precision float=w137:dbl)
            n142 = property on="sample" class="Slide (strict)"("Scale.Maximum"=w133) -> ()  [unwired: 2 in, 2 out]
            n143 = property on="block" class="Slide (strict)"("Scale.Maximum"=w131) -> ()  [unwired: 2 in, 2 out]
            n144 = Multiply(x=w142, y=w137) -> (x*y=→"MB RAM":dbl)
            n145 = global write "Globals.vi" "nos"("no.of samples (nos)") -> ()
            n146 = Multiply(x="no.of samples (nos)", y="no.of blocks (nob)\npress enter") -> (x*y=w135:u32)
            n147 = global write "Globals.vi" "nob"("no.of blocks (nob)\npress enter") -> ()
            n148 = To Double Precision Float(number=w135) -> (double precision float=w136:dbl)
            n149 = global write "Globals.vi" "exp time"("exposuretime[ms]") -> ()
            n150 = Multiply(x="exposuretime[ms]", y=w136) -> (x*y=w148:dbl)
            n151 = Divide(x=w148, y=1000.0) -> (x/y=→"SEC":dbl)
          }
          event "stop all": Value Change {
            # "exit"
            n152 = event-data() -> ()  [unwired: 1 in, 6 out]
            n153 = stacked-sequence {
              tunnel: [_ TRUE] -> w153
              frame #0 {
                n154 = call "FFStop.vi"() -> ()  [unwired: 1 in]
              }
              frame #1 {
                # "do not omit, or next call of driver will go wrong."
                n155 = call "Exit.vi"() -> ()  [unwired: 1 in]
              }
            }
          }
          event "rms_pixel": Value Change {
            # "one array with all values (except first 10)\nat index Pixel from all blocks"
            n156 = event-data() -> ()  [unwired: 1 in, 6 out]
            n157 = global read "Globals.vi" "nos"() -> (w159:u32)
            n158 = global read "Globals.vi" "nob"() -> (w160:u32)
            n159 = for {
              N: w160 -> [_]
              tunnel: w159 -> [w161]
              tunnel: [w163] -> w156 mode=concatenating
              i -> [w167]
              # "delete first 10 values"
              # "array of all values\nat index Pixel"
              n160 = To Long Integer(number=w161) -> (32bit integer=w162:i32)
              n161 = for {
                N: w162 -> [_]
                tunnel: w167 -> [w172]
                tunnel: [w176] -> w164 mode=indexing
                i -> [w174]
                # "use only value at index \"Pixel\""
                # "init array of size PIXEL\nwith value 100"
                n162 = global read "Globals.vi" "PIXEL"() -> (w168:u32)
                n163 = To Long Integer(number=w168) -> (32bit integer=w169:i32)
                n164 = To Unsigned Long Integer(number=w172) -> (unsigned 32bit integer=w173:u32)
                n165 = To Unsigned Long Integer(number=w174) -> (unsigned 32bit integer=w175:u32)
                n166 = Initialize Array(u16 100, w169) -> (w178:u16[])
                n167 = call "ReturnFrame.vi"("Data Values In"=w178, "curr_nob"=w173, "curr_nos"=w175, "Drv"=u32 1) -> ("Data Values Out"=w177:u16[])  [unwired: 1 in]
                n168 = To Long Integer(number="rms_pixel") -> (32bit integer=w170:i32)
                n169 = Index Array(array=w177, index=w170) -> (element=w176:u16)
              }
              n170 = Delete From Array(array=w164, length=10, index=0) -> (array with subset deleted=w163:u16[])  [unwired: 1 out]
            }
            n171 = To Double Precision Float(number=w156) -> (double precision float=w155:dbl[])
            n172 = call <vilib>:"Std Deviation and Variance.vi"("X"=w155) -> ("mean"=→"mean":dbl, "standard deviation"=→"tRMS":dbl)  [unwired: 1 in, 1 out]
          }
          event "ADC mode": Value Change {
            n173 = event-data() -> ()  [unwired: 1 in, 6 out]
            n174 = case shown="\"3\"" "ADC mode" {
              frame "1" {
                w182 = u16 0  # data
                w183 = u8 38  # adadr
                w184 = u8 1  # madr
                w185 = u16 18  # data
                w186 = u8 37  # adadr
                w187 = u8 1  # madr
                # "Custom Pattern"
                n175 = call "SendFLCam.vi"("madr"=w187, "data"=w185, "adadr"=w186) -> ()
                n176 = call "SendFLCam.vi"("madr"=w184, "data"=w182, "adadr"=w183) -> ()
              }
              frame "2" {
                w188 = u16 64  # data
                w189 = u8 37  # adadr
                w190 = u8 1  # madr
                # "Ramp"
                n177 = call "SendFLCam.vi"("madr"=w190, "data"=w188, "adadr"=w189) -> ()
              }
              frame "3" {
                w191 = u16 1  # data
                w193 = u8 0  # adadr
                w192 = u8 1  # madr
                w196 = u16 0  # data
                w195 = u8 38  # adadr
                w194 = u8 1  # madr
                w199 = u16 0  # data
                w198 = u8 37  # adadr
                w197 = u8 1  # madr
                # "Normal Mode"
                n178 = call "SendFLCam.vi"("madr"=w194, "data"=w196, "adadr"=w195) -> ()
                n179 = call "SendFLCam.vi"("madr"=w192, "data"=w191, "adadr"=w193) -> ()
                n180 = call "SendFLCam.vi"("madr"=w197, "data"=w199, "adadr"=w198) -> ()
              }
            }
          }
        }
      }
    }
  }
  n181 = property on="sample" class="Slide (strict)"("DisabledEnum"=w1) -> ()  [unwired: 2 in, 2 out]
  n182 = property on="start" class="Bool (strict)"("DisabledEnum"=w1) -> ()  [unwired: 2 in, 2 out]
  n183 = property on="block" class="Slide (strict)"("DisabledEnum"=w1) -> ()  [unwired: 2 in, 2 out]
